vi "DMSC.ShutDownCommand.vi"(1 "SD_DMS":refnum<user-event>, 3 "SDConnection Event":refnum<user-event>) -> ()   [LabVIEW 2014, in "DMSClient.lvlib"]
uses:
  DMSClient.lvlib
  <resource>/objmgr/ni.dex.rc
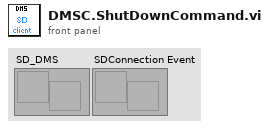
[diagram p1: front panel]
types:
  T1 = cluster{"SystemName":string, "SDWriterEP":refnum<k21>, "ConStatus":enum16{"Init", "Comm"}}[]
  T2 = cluster{"SystemName":string, "SDWriterEP":refnum<k21>, "ConStatus":enum16{"Init", "Comm"}}
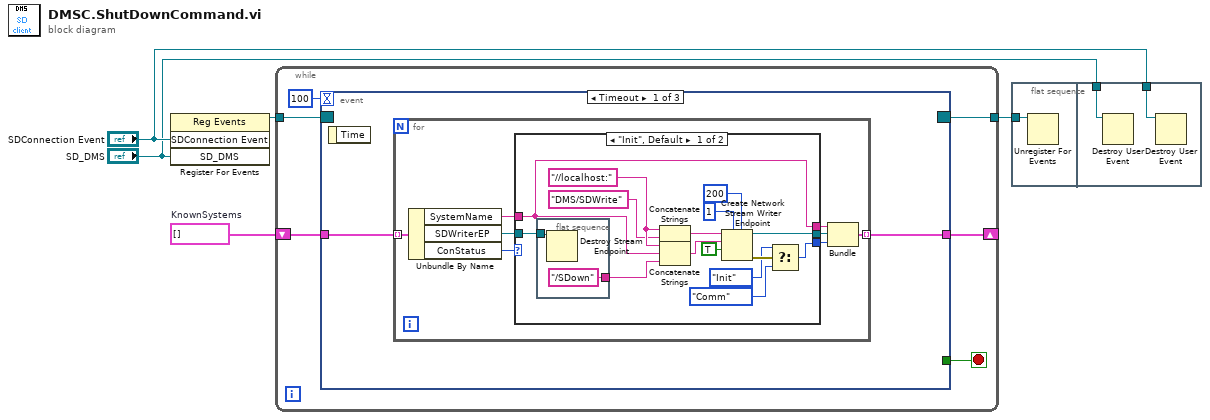
[diagram p0: block diagram]
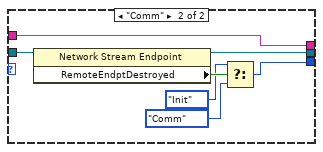
[diagram p2: hidden frame]
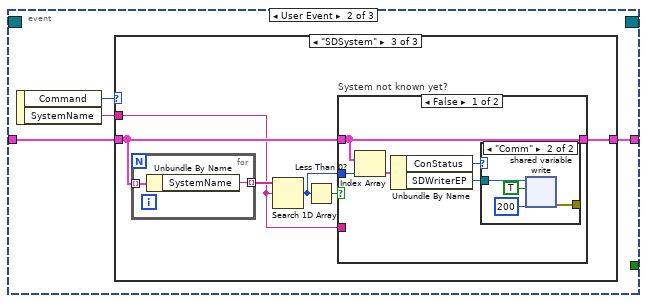
[diagram p3: hidden frame]
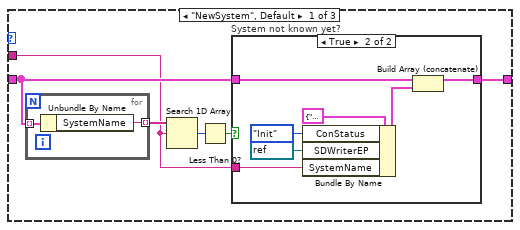
[diagram p4: hidden frame]
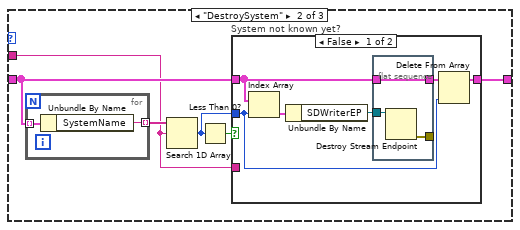
[diagram p6: hidden frame]
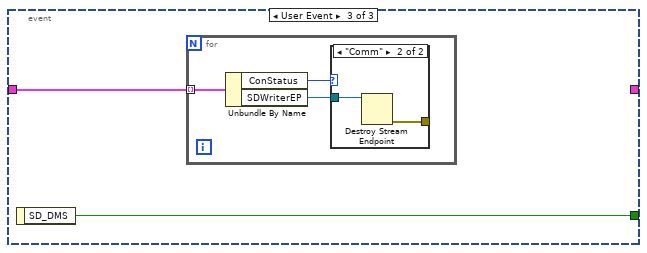
[diagram p10: hidden frame]
diagram:
  w4 = T1 []  # KnownSystems
  n1 = register-events("SDConnection Event", "SD_DMS") -> (reference out=w5:refnum<event-registration>)  [unwired: 2 in, 1 out]
  n2 = while {
    tunnel: w5 -> [w11]
    shift-right: [w8] -> _
    shift-left: w4 -> [w9]
    tunnel: [w6] -> w3
    stop <- w7 stop-if-true
    n3 = event shown="[0] Timeout" {
      selector: w11 -> [_ _ _]
      dyn-events: [_ _ _] -> w6
      timeout: 100 -> [_ _ _]
      tunnel: w9 -> [w13 w47 w102]
      tunnel: [w12 w46 _] -> w8
      tunnel: [_ _ w103] -> w7
      event Timeout {
        n4 = event-data() -> ()  [unwired: 1 in, 1 out]
        n5 = for {
          tunnel: w13 -> [w21] mode=indexing
          tunnel: [w17] -> w12 mode=indexing
          n6 = Unbundle By Name(w21) -> ("SystemName"=w18:string, "SDWriterEP"=w19:refnum<k21>, "ConStatus"=w20:enum16{"Init", "Comm"})
          n7 = case shown="\"Init\", Default" w20 {
            tunnel: w19 -> [w36 w45]
            tunnel: w18 -> [w24 w39]
            tunnel: [w28 w41] -> w16
            tunnel: [w32 w40] -> w15
            tunnel: [w24 w39] -> w14
            frame "Init", Default {
              w25 = "//localhost:" ("string")
              n8 = flat-sequence {
                tunnel: w36 -> [w38]
                tunnel: ["/SDown" ("string")] -> w23
                frame #0 {
                  n9 = Destroy Stream Endpoint(11:w38) -> ()  [unwired: 1 in, 1 out]
                }
              }
              n10 = Concatenate Strings(w25, "DMS/SDWrite" ("string")) -> (w27:string)
              n11 = Concatenate Strings(w25, w24, w23) -> (w26:string)
              n12 = Create Network Stream Writer Endpoint(5:200 ("timeout in ms (-1)"), 7:1 ("writer buffer size"), 9:TRUE, 10:w26, 11:w27) -> (0:w31:errorcluster, 3:w32:refnum<k21>)  [unwired: 2 in]
              n13 = Select(t=enum16{"Init", "Comm"}."Init" ("ConStatus"), s=w31, f=enum16{"Init", "Comm"}."Comm" ("ConStatus")) -> (s? t:f=w28:enum16{"Init", "Comm"})
            }
            frame "Comm" {
              n14 = property class="Network Stream Endpoint"(reference=w45) -> (reference out=w40:refnum<k21>, "RemoteEndptDestroyed"=w44:bool)  [unwired: 1 in, 1 out]
              n15 = Select(t=enum16{"Init", "Comm"}."Init" ("ConStatus"), s=w44, f=enum16{"Init", "Comm"}."Comm" ("ConStatus")) -> (s? t:f=w41:enum16{"Init", "Comm"})
            }
          }
          n16 = Bundle("SystemName"=w14, "SDWriterEP"=w15, "ConStatus"=w16) -> (w17:T2)  [unwired: 1 in]
        }
      }
      event User Event {
        n17 = event-data() -> ("Command"=w49:enum16{"NewSystem", "DestroySystem", "SDSystem"}, "SystemName"=w48:string)  [unwired: 1 in]
        n18 = case shown="\"SDSystem\"" w49 {
          tunnel: w48 -> [w50 w67 w85]
          tunnel: w47 -> [w52 w69 w87]
          tunnel: [w51 w68 w86] -> w46
          frame "NewSystem", Default {
            n19 = for {
              tunnel: w52 -> [w65] mode=indexing
              tunnel: [w64] -> w55 mode=indexing
              n20 = Unbundle By Name(w65) -> ("SystemName"=w64:string)
            }
            n21 = Search 1D Array(1D array=w55, element=w50) -> (index of element=w54:i32)  [unwired: 1 in]
            n22 = Less Than 0?(x=w54) -> (x < 0?=w53:bool)
            n23 = case "System not known yet?" shown="True" w53 {
              tunnel: w52 -> [w56 w63]
              tunnel: [w56 w62] -> w51
              tunnel: w50 -> [_ w60]
              frame False {
              }
              frame True {
                n24 = Bundle By Name(cluster=T2 {"SystemName"="", "SDWriterEP"="", "ConStatus"=enum."Init"}, "ConStatus"=enum16{"Init", "Comm"}."Init", "SDWriterEP"=refnum<k21> refnum, "SystemName"=w60) -> (w61:T2)
                n25 = Build Array (concatenate)(w63, w61) -> (w62:T1)
              }
            }
          }
          frame "DestroySystem" {
            n26 = for {
              tunnel: w69 -> [w83] mode=indexing
              tunnel: [w82] -> w71 mode=indexing
              n27 = Unbundle By Name(w83) -> ("SystemName"=w82:string)
            }
            n28 = Search 1D Array(1D array=w71, element=w67) -> (index of element=w66:i32)  [unwired: 1 in]
            n29 = Less Than 0?(x=w66) -> (x < 0?=w70:bool)
            n30 = case "System not known yet?" shown="False" w70 {
              tunnel: w69 -> [w75 w81]
              tunnel: [w73 w81] -> w68
              tunnel: w67 -> [_ _]
              tunnel: w66 -> [w72 _]
              frame False {
                n31 = Index Array(array=w75, index=w72) -> (element=w77:T2)
                n32 = Unbundle By Name(w77) -> ("SDWriterEP"=w76:refnum<k21>)
                n33 = flat-sequence {
                  tunnel: w76 -> [w80]
                  tunnel: w75 -> [w78]
                  tunnel: [w79] -> _
                  tunnel: [w78] -> w74
                  frame #0 {
                    n34 = Destroy Stream Endpoint(11:w80) -> (0:w79:errorcluster)  [unwired: 1 in]
                  }
                }
                n35 = Delete From Array(array=w74, index=w72) -> (array with subset deleted=w73:T1)  [unwired: 1 in, 1 out]
              }
              frame True {
              }
            }
          }
          frame "SDSystem" {
            n36 = for {
              tunnel: w87 -> [w101] mode=indexing
              tunnel: [w100] -> w89 mode=indexing
              n37 = Unbundle By Name(w101) -> ("SystemName"=w100:string)
            }
            n38 = Search 1D Array(1D array=w89, element=w85) -> (index of element=w84:i32)  [unwired: 1 in]
            n39 = Less Than 0?(x=w84) -> (x < 0?=w88:bool)
            n40 = case "System not known yet?" shown="False" w88 {
              tunnel: w87 -> [w93 w99]
              tunnel: [w93 w99] -> w86
              tunnel: w85 -> [_ _]
              tunnel: w84 -> [w94 _]
              frame False {
                n41 = Index Array(array=w93, index=w94) -> (element=w92:T2)
                n42 = Unbundle By Name(w92) -> ("ConStatus"=w91:enum16{"Init", "Comm"}, "SDWriterEP"=w90:refnum<k21>)
                n43 = case shown="\"Comm\"" w91 {
                  tunnel: w90 -> [_ w97]
                  tunnel: [_ w96] -> _
                  frame "Init", Default {
                  }
                  frame "Comm" {
                    n44 = shared-variable-write(w97, TRUE, 200 ("timeout ms (-1)")) -> (w96:errorcluster)  [unwired: 1 in, 2 out]
                  }
                }
              }
              frame True {
              }
            }
          }
        }
      }
      event User Event {
        n45 = event-data() -> ("SD_DMS"=w103:bool)  [unwired: 1 in]
        n46 = for {
          tunnel: w102 -> [w106] mode=indexing
          n47 = Unbundle By Name(w106) -> ("ConStatus"=w105:enum16{"Init", "Comm"}, "SDWriterEP"=w104:refnum<k21>)
          n48 = case shown="\"Comm\"" w105 {
            tunnel: w104 -> [_ w108]
            tunnel: [_ w107] -> _
            frame "Init", Default {
            }
            frame "Comm" {
              n49 = Destroy Stream Endpoint(11:w108) -> (0:w107:errorcluster)  [unwired: 1 in]
            }
          }
        }
      }
    }
  }
  n50 = flat-sequence {
    tunnel: w3 -> [w109]
    tunnel: "SDConnection Event" -> [w111]
    tunnel: "SD_DMS" -> [w110]
    frame #0 {
      n51 = Unregister For Events(event registration refnum=w109) -> ()  [unwired: 1 in, 1 out]
    }
    frame #1 {
      n52 = Destroy User Event(user event=w110) -> ()  [unwired: 1 in, 1 out]
      n53 = Destroy User Event(user event=w111) -> ()  [unwired: 1 in, 1 out]
    }
  }
